vi "Command Settings.vi"() -> (5 "Command Stats":cluster{"Enum":T1, "U8":u8, "Payload":bool}[](array[cluster])=[{"Enum"=enum."Status", "U8"=0, "Payload"=TRUE}])   [LabVIEW 2021, in "CIFTemplateCoreOOB_Tx.lvclass"]
uses:
  CIFTemplateCoreOOB_Tx.lvclass
  Typedef/OOB Core Commands.ctl
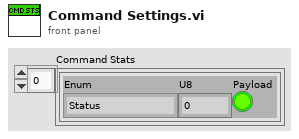
[diagram p1: front panel]
types:
  T1 = typedef "CIFTemplateCoreOOB_Tx.lvclass/OOB Core Commands.ctl" = enum8{"Status"}
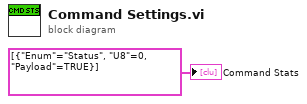
[diagram p0: block diagram]
diagram:
  "Command Stats" <- cluster{"Enum":T1, "U8":u8, "Payload":bool}[] [{"Enum"=enum."Status", "U8"=0, "Payload"=TRUE}]
